vi "Write File Permission Parameters.vi"(0 "PDF Report Class in":refnum<class "PDF Report Class.lvclass">, 7 "File Permission Parameters":T1={"User Password"="", "Owner Password"="", "Printing"=enum."Allow Printing", "Allow Modify Contents"=FALSE, "Allow Copy"=FALSE, "Allow Modify Annotations"=TRUE, "Allow Fill In "=TRUE, "Allow Screen Readers"=FALSE, "Allow Assembly"=FALSE}, 11 "error in (no error)":errorcluster) -> (4 "PDF Report Class out":refnum<class "PDF Report Class.lvclass">, 15 "error out":errorcluster)   [LabVIEW 2019, in "Exaprom PDF.lvlib" / "PDF Report Class.lvclass"]
uses:
  PDF Report Class.lvclass
  Controls/Initialization Controls/File Permission Parameters.ctl
  PDF Report Class.lvclass/PDF Report Class.ctl
  Exaprom PDF.lvlib
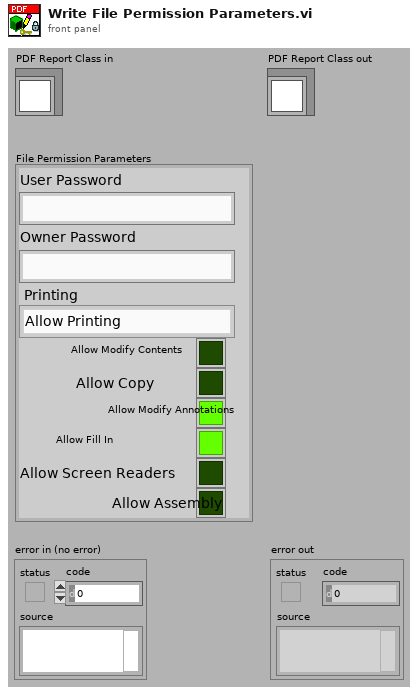
[diagram p1: front panel]
types:
  T1 = typedef "Exaprom PDF.lvlib/File Permission Parameters.ctl" = cluster{"User Password":string, "Owner Password":string, "Printing":enum16{"Allow Printing", "Allow Degraded Printing", "Don't Allow Printing"}, "Allow Modify Contents":bool, "Allow Copy":bool, "Allow Modify Annotations":bool, "Allow Fill In ":bool, "Allow Screen Readers":bool, "Allow Assembly":bool}
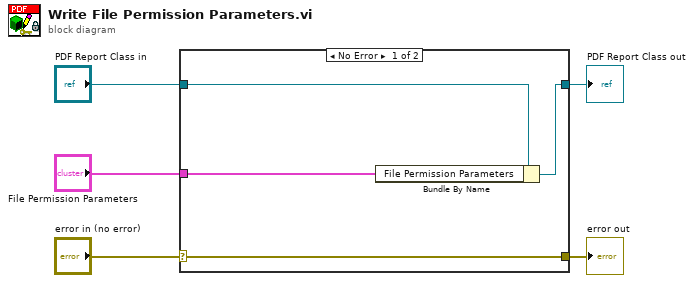
[diagram p0: block diagram]
diagram:
  n1 = case shown="No Error" "error in (no error)" {
    selector: "error in (no error)" -> [w9 w10]
    tunnel: [w9 w10] -> w4
    tunnel: [w7 w11] -> w2
    tunnel: "PDF Report Class in" -> [w8 w11]
    tunnel: "File Permission Parameters" -> [w6 _]
    frame No Error {
      n2 = Bundle By Name(cluster=w8, "File Permission Parameters"=w6) -> (w7:refnum<class "PDF Report Class.lvclass">)
    }
    frame Error {
    }
  }
  "error out" <- w4
  "PDF Report Class out" <- w2
